vi "DistToObstNearwAng.vi"(9 "Boat Point":T1 {"North" format="%#_10f"; "East" format="%#_8f"}, 10 "Segment Point 2":T1 {"North" format="%#_10f"; "East" format="%#_8f"}, 11 "Segment Point 1":T1 {"North" format="%#_10f"; "East" format="%#_8f"}) -> (2 "Angle to Obstacle, Trig Abs":dbl, 3 "Distance between boat and segment":dbl)   [LabVIEW 2013]
doc: "Takes in a segment, and a boat point, and returns the distance between the segment and the boat. For obstacle avoidance. To be added: absolute trig angle to segment."
uses:
  Data/TypeDefs/UTM Location.ctl
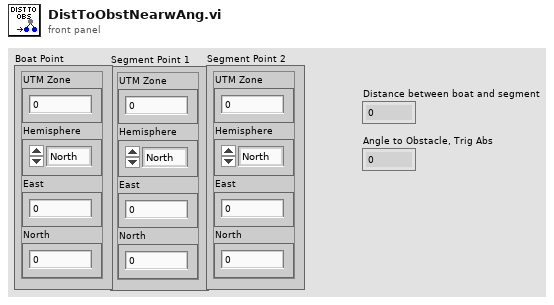
[diagram p1: front panel]
types:
  T1 = typedef "UTM Location.ctl" = cluster{"UTM Zone":dbl, "Hemisphere":enum16{"North", "South"}, "East":dbl, "North":dbl}
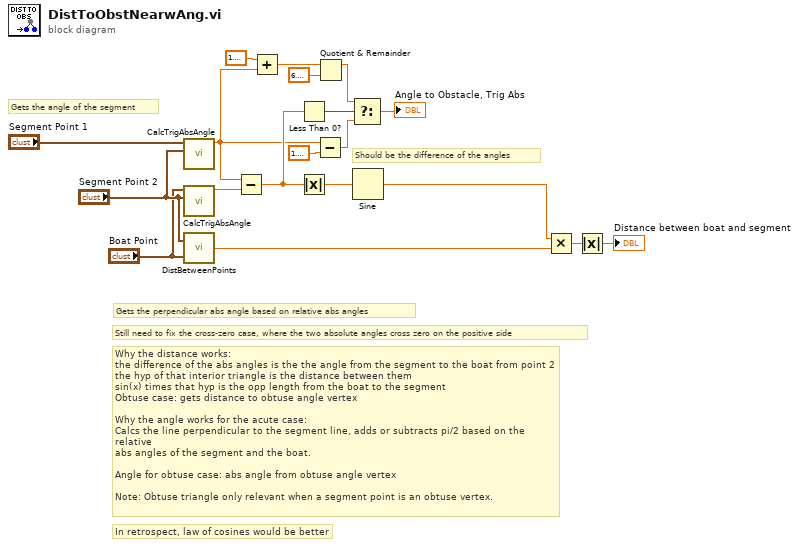
[diagram p0: block diagram]
diagram:
  # "In retrospect, law of cosines would be better"
  # "Gets the perpendicular abs angle based on relative abs angles"
  # "Still need to fix the cross-zero case, where the two absolute angles cross zero on the positive side"
  # "Why the distance works:\nthe difference of the abs angles is the the angle from the segment to the boat from point 2\nthe hyp of that interior triangle is the distance between them\nsin(x) times that hyp is the opp length from the boat to the segment\nObtuse case: gets distance to obtuse angle vertex\n\nWhy the angle works for the acute case:\nCalcs the line perpendicular to the segment line, adds or subtracts pi/2 based on the relative\nabs angles of the segment and the boat.\n\nAngle for obtuse case: abs angle from obtuse angle vertex \n\nNote: Obtuse triangle only relevant when a segment point is an obtuse vertex."
  # "Should be the difference of the angles"
  # "Gets the angle of the segment"
  n1 = call "CalcTrigAbsAngle.vi"("Point 2"="Segment Point 2", "Point 1"="Segment Point 1") -> ("Angle between points (rad)"=w7:dbl)  [unwired: 9 in]
  n2 = call "CalcTrigAbsAngle.vi"("Point 2"="Segment Point 2", "Point 1"="Boat Point") -> ("Angle between points (rad)"=w19:dbl)  [unwired: 9 in]
  n3 = call "DistBetweenPoints.vi"("UTM Location 2"="Boat Point", "UTM Location"="Segment Point 2") -> ("Numeric"=w18:dbl)
  n4 = Subtract(x=w7, y=w19) -> (x-y=w8:dbl)
  n5 = Add(x=1.5707963267948966, y=w7) -> (x+y=w4:dbl)
  n6 = Less Than 0?(x=w8) -> (x < 0?=w13:bool)
  n7 = Absolute Value(x=w8) -> (abs(x)=w3:dbl)
  n8 = Subtract(x=w7, y=1.5707963267948966) -> (x-y=w12:dbl)
  n9 = Quotient & Remainder(x=w4, y=6.283185307179586) -> (x-y*floor(x/y)=w6:dbl)  [unwired: 1 out]
  n10 = Select(t=w6, s=w13, f=w12) -> (s? t:f=→"Angle to Obstacle, Trig Abs":dbl)
  n11 = Sine(x=w3) -> (sin(x)=w17:dbl)
  n12 = Multiply(x=w17, y=w18) -> (x*y=w16:dbl)
  n13 = Absolute Value(x=w16) -> (abs(x)=→"Distance between boat and segment":dbl)
